vi "ProceedProcessSelection.vi"(8 "Error In":errorcluster, 10 "Selected Param":variant, 11 "MulticolumnListbox in":refnum<vi>) -> (0 "error out":errorcluster)   [LabVIEW 2019]
uses:
  Controls/ProcessDataEntry_Action.ctl
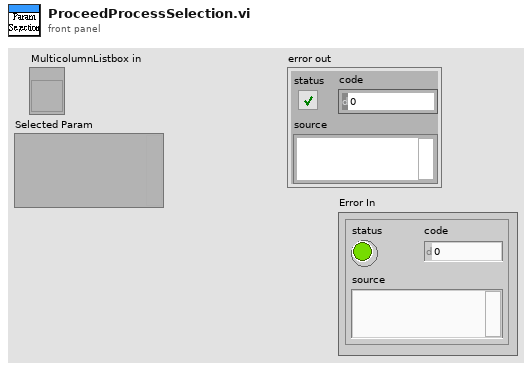
[diagram p1: front panel]
types:
  T1 = typedef "ProcessDataEntry_Action.ctl" = enum16{"Intial", "UpdateSteps", "ReallAllSteps", "ReadStep"}
  T2 = typedef "Process_Setting.ctl" = cluster{"Enum_PreProcess":T3, "Parameter":string}
  T3 = typedef "VisionProcessName.ctl" = enum16{"*CamParameter*", "CamAttributes", "*Preprocess*", "CG_Brightness", "C_Plane Extraction", "C_Threshold", "G_Lookup Table", "G_Threshold"}
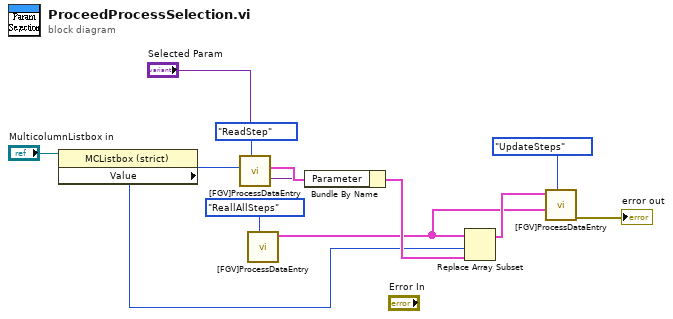
[diagram p0: block diagram]
diagram:
  n1 = property on="Property Node" class="MCListbox (strict)"(reference="MulticolumnListbox in") -> ("Value"=w7:i32)  [unwired: 1 in, 2 out]
  n2 = call "[FGV]ProcessDataEntry.vi"("ProcessDataEntry_Action"=ProcessDataEntry_Action."ReadStep", "Prcocess Step"=w7) -> ("ProcessSetting Out"=w6:T2)  [unwired: 6 in, 3 out]
  n3 = call "[FGV]ProcessDataEntry.vi"("ProcessDataEntry_Action"=ProcessDataEntry_Action."ReallAllSteps") -> ("AllProcessSettingOut"=w1:T2[])  [unwired: 7 in, 3 out]
  n4 = Bundle By Name(cluster=w6, "Parameter"="Selected Param") -> (w8:T2)
  n5 = Replace Array Subset(array=w1, new element=w8, index=w7) -> (w10:T2[])
  n6 = call "[FGV]ProcessDataEntry.vi"("ProcessDataEntry_Action"=ProcessDataEntry_Action."UpdateSteps", "OldAllProcessSetting In"=w1, "AllProcessSetting In"=w10) -> ("Error Out"=→"error out":errorcluster)  [unwired: 5 in, 3 out]
